vi "AlliGator Image Profile Menu Check Marks.vi"(8 "Error In":errorcluster, 11 "Menu in":refnum<k9>) -> (0 "Error Out":errorcluster)   [LabVIEW 2021, in "AlliGator Image Profile Window.lvlib"]
doc: "Handles checked items in Profile Window menu."
uses:
  AlliGator Image Profile Window.lvlib
  AlliGator Variables List.ctl
  Image/Box Profile Type.ctl
  AlliGator Image Profile Intensity Type.ctl
  AlliGator Image Profile Average Intensity Type.ctl
  Variant/Variant to Data/Variant to Boolean.vi
  AlliGator Globals, Variables & Constants.lvlib
  Variant/Variant to Data/Variant to Data.lvlib
  Image/Image.lvlib
panel:
  # "see the AlliGator License on the block diagram (Ctrl+E or Window:Show Block Diagram)"
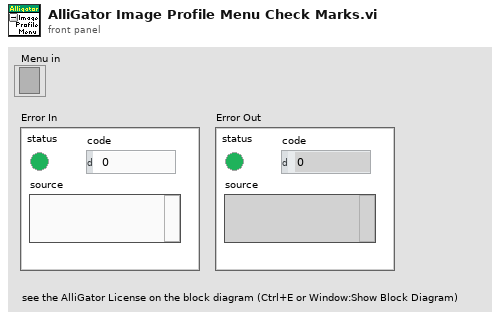
[diagram p1: front panel]
types:
  T1 = typedef "AlliGator Image Profile Window.lvlib/AlliGator Image Profile Average Intensity Type.ctl" = enum16{"Integrated Intensity", "Average Intensity", "Intensity-weighted Average Intensity"}
  T2 = typedef "AlliGator Image Profile Window.lvlib/AlliGator Image Profile Intensity Type.ctl" = enum16{"Raw Data", "Displayed Image", "Background-subtracted"}
  T3 = typedef "AlliGator Globals, Variables & Constants.lvlib/AlliGator Variables List.ctl" = enum16{"---- GUI ----", "Initialization Status", "State Indicators Refnum", "Original AlliGator Menu Items", "Current Action Loop State", "Script in progress", "Playback", "Loop Playback", "Search ROI Used", "Search ROI", "Decay Graph Max Legend Size", "Intensity Graph Max Legend Size", "Decay Statistics Graph Max Legend Size", "Phasor Graph Max Legend Size", "Phasor Ratio Graph Max Legend Size", "Lifetime Graph Max Legend Size", "---- Files ----", "Export Dataset Frames as Individual Files", "Show Batch Export Help Balloons", "Frames in Dataset", "ptu File Frame Start Indices", "Current Frame in Dataset", "Current Frame Timestamp", "------ Python Plugins ------", "Python Plugins Information", "Python Session", "Valid Python Session?", "---- Source Image ----", "Dataset Loaded", "Dataset Metadata", "Dataset Channel", "Dataset Data Description", "Background Dataset Metadata", "Background Dataset Channel", "Background Dataset Data Description", "Background File Subtraction", "Background File Path", "Background File Pile-up Correction", "Background File Pixel Well Capacity", "Background File Scaling Factor", "Source Image ROIs", "Current Source Image ROI", "Source Image ROI Event Refnum", "X_Source Image Display Range", "X_Source Image Palette Information", "Source Image Palette List", "Source Image Scale", "Current Dataset Load Settings", "Source Image:ROI Overlay Color", "---- Image Profile Window ----", "Image Profile:Overlay ROI in Source Image", "Image Profile Window Event Refnum", "Image Profile:IntensityType", "Image Profile:Intensity Average Type", "Image Profile:Intensity-weighted SDV", "Image Profile:Box Profile Type", "Image Profile Window Open", "Image Profile:Plotted Fit Parameter", "X_Type of Displayed Image", "X_Time Gate Slider", "Dataset Path", "Source Image Overlay to Erase", "Is Displayed Image Accumulated", "White Light Image Modified", "Mask Image Modified", "Macrotime Gate Separation", "------ Phasor Graph -------", "Phasor Graph:Show Line", "---- Phasor Plot ---", "Phasor Plot Parameters Changed", "FLI Dataset Modified since last Phasor Plot Calculation", "Phasor Harmonics Data", "Selected Phasor Harmonics", "Phasor Harmonic Manager Event Refnum", "Phasor Plot ROIs", "Current Phasor Plot ROI", "Phasor Plot ROI Event Refnum", "Phasor Plot Image Reference Points", "Phasor Plot Computed", "Phasor Plot Palette Information", "Phasor Plot Palette List", "Phasor Ratio Palette Information", "Phasor Ratio Palette List", "Phasor Image Scale", "Phasor Plot Image Overlay to Erase", "Phasor Plot Image Elements to Update", "Current Phasor Plot Calculation Parameters", "Current Phasor Calibration Options", "Reset Cumulated Phasor Plot", "Phasor Ratio Reference 1", "Phasor Ratio Lifetime Reference 1", "Phasor Ratio Reference 1 Frequency", "Phasor Ratio Reference 2", "Phasor Ratio Lifetime Reference 2", "Phasor Ratio Reference 2 Frequency", "---- Decay Analysis ----", "Number of Selected Decays to Fit", "LS Fit Results", "LAR Fit Results", "BS Fit Results", "Last Decay Max - Min", "Best Fit Parameters", "Best Fit Parameter Names", "Actual Size X", "Actual Size Y", "Binning X", "Binning Y", "Actual # Gates", "Dataset Number", "Gates to...", "Gates Skipped", "Gates to keep", "Gate Step", "Gate Separation", "Reversed Gates", "Pile-up Correction", "Pixel Well Capacity", "Background Subtracted", "Background Subtraction Method", "Background Definition Range", "Background File (deprecated)", "Number of Dataset Accumulated", "Array of Accumulated Dataset Paths", "Do Averaged Datasets", "Destination File Path", "Process Plot Target", "Use 1/D as Phasor Frequency", "---- Decay Fit Parameter Map -----", "Decay Fit Parameter Map Palette Information", "Decay Fit Parameter Map Palette List", "Local Decay Graph Window Event Refnum", "------- Local Decay Window ---------", "Use normalized IRF for convolution", "----- Miscellaneous ----", "Skippable Dialog Windows Status"}
  T4 = typedef "Image.lvlib/Box Profile Type.ctl" = enum16{"Full Width", "Half Width"}
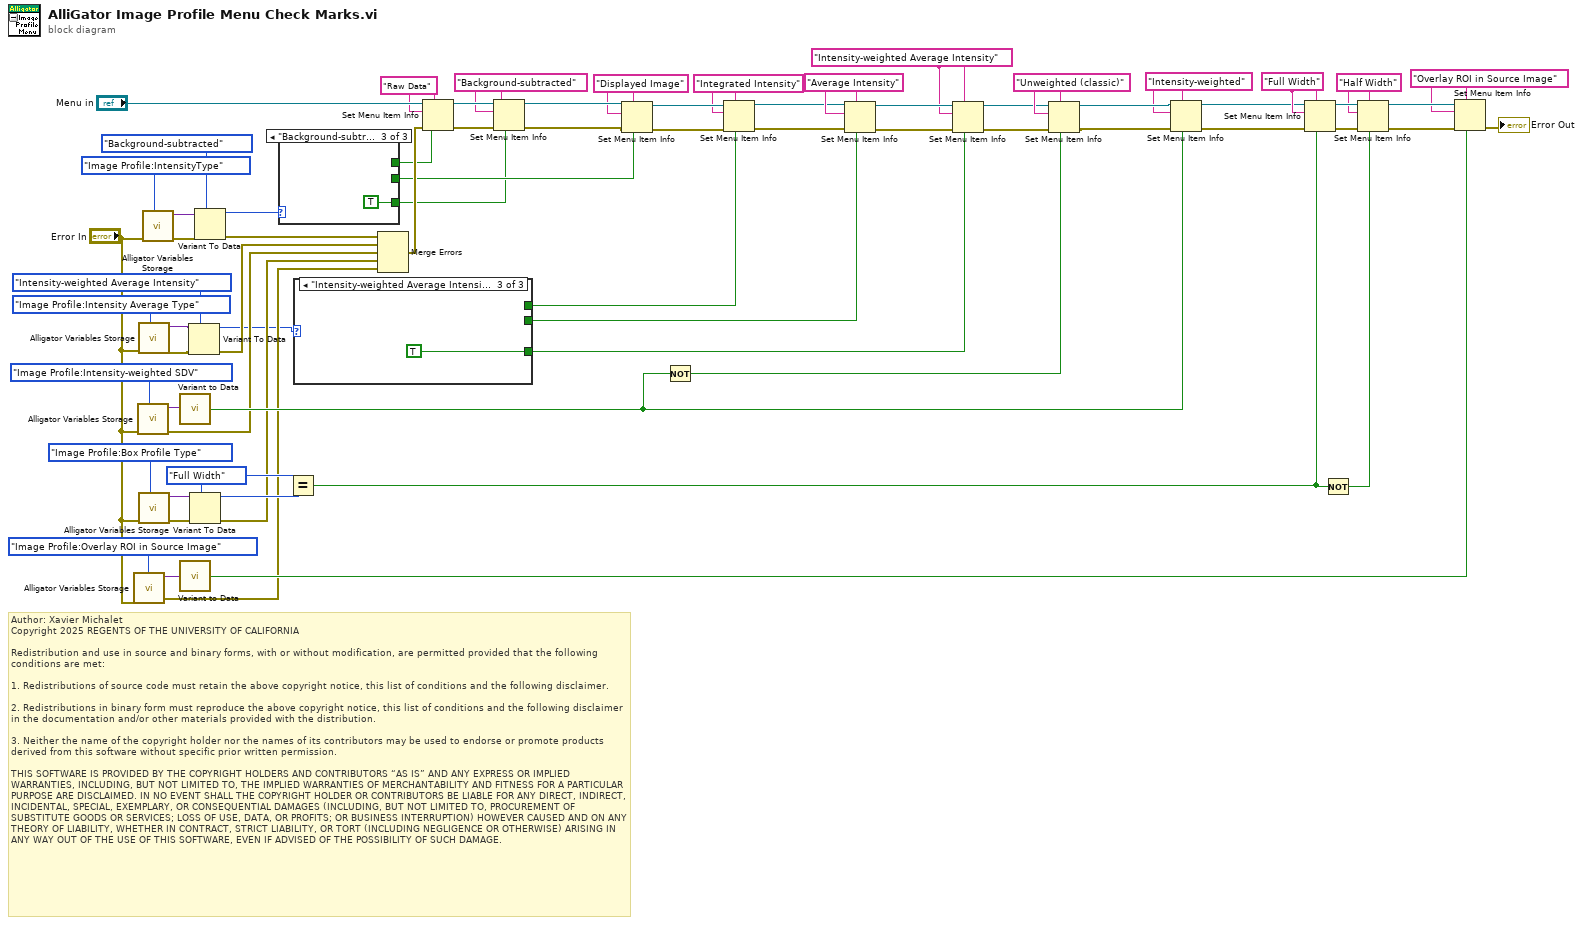
[diagram p0: block diagram]
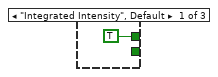
[diagram p2: hidden frame]
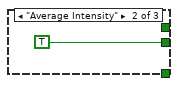
[diagram p3: hidden frame]
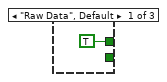
[diagram p4: hidden frame]
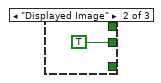
[diagram p5: hidden frame]
diagram:
  w2 = "Integrated Intensity" ("ItemTag")
  w9 = "Intensity-weighted Average Intensity" ("ItemTag")
  w10 = "Average Intensity" ("ItemTag")
  w30 = "Overlay ROI in Source Image" ("item tag")
  w46 = "Half Width" ("item tag")
  w44 = "Full Width" ("item tag")
  w48 = Box_Profile_Type."Full Width"
  w53 = "Intensity-weighted" ("ItemTag")
  w58 = "Unweighted (classic)" ("ItemTag")
  w61 = "Displayed Image" ("ItemTag")
  w65 = "Background-subtracted" ("ItemTag")
  w67 = "Raw Data" ("ItemTag")
  # "Author: Xavier Michalet\nCopyright 2025 REGENTS OF THE UNIVERSITY OF CALIFORNIA\n\nRedistribution and use in source and binary forms, with or without modification, are permitted provided that the following conditions are met:\n\n1. Redistributions of source code must retain the above copyright notice, this list of conditions and the following disclaimer.\n\n2. Redistributions in binary form must reproduce the above copyright notice, this list of conditions and the following disclaimer in the documentation and/or other materials provided with the distribution.\n\n3. Neither the name of the copyright holder nor the names of its contributors may be used to endorse or promote products derived from this software without specific prior written permission.\n\nTHIS SOFTWARE IS PROVIDED BY THE COPYRIGHT HOLDERS AND CONTRIBUTORS “AS IS” AND ANY EXPRESS OR IMPLIED WARRANTIES, INCLUDING, BUT NOT LIMITED TO, THE IMPLIED WARRANTIES OF MERCHANTABILITY AND FITNESS FOR A PARTICULAR PURPOSE ARE DISCLAIMED. IN NO EVENT SHALL THE COPYRIGHT HOLDER OR CONTRIBUTORS BE LIABLE FOR ANY DIRECT, INDIRECT, INCIDENTAL, SPECIAL, EXEMPLARY, OR CONSEQUENTIAL DAMAGES (INCLUDING, BUT NOT LIMITED TO, PROCUREMENT OF SUBSTITUTE GOODS OR SERVICES; LOSS OF USE, DATA, OR PROFITS; OR BUSINESS INTERRUPTION) HOWEVER CAUSED AND ON ANY THEORY OF LIABILITY, WHETHER IN CONTRACT, STRICT LIABILITY, OR TORT (INCLUDING NEGLIGENCE OR OTHERWISE) ARISING IN ANY WAY OUT OF THE USE OF THIS SOFTWARE, EVEN IF ADVISED OF THE POSSIBILITY OF SUCH DAMAGE."
  n1 = call "Alligator Variables Storage.vi"("AlliGator Variable"=AlliGator_Variables_List."Image Profile:Overlay ROI in Source Image" ("Alligator Variable"), "Error In"="Error In") -> ("Error Out"=w31:errorcluster, "Data out"=w36:variant)  [unwired: 7 in, 1 out]
  n2 = call "Alligator Variables Storage.vi"("AlliGator Variable"=AlliGator_Variables_List."Image Profile:Intensity-weighted SDV" ("Alligator Variable"), "Error In"="Error In") -> ("Error Out"=w38:errorcluster, "Data out"=w59:variant)  [unwired: 7 in, 1 out]
  n3 = call "Alligator Variables Storage.vi"("AlliGator Variable"=AlliGator_Variables_List."Image Profile:Intensity Average Type" ("Alligator Variable"), "Error In"="Error In") -> ("Error Out"=w19:errorcluster, "Data out"=w18:variant)  [unwired: 7 in, 1 out]
  n4 = call "Alligator Variables Storage.vi"("AlliGator Variable"=AlliGator_Variables_List."Image Profile:Box Profile Type" ("Alligator Variable"), "Error In"="Error In") -> ("Error Out"=w50:errorcluster, "Data out"=w51:variant)  [unwired: 7 in, 1 out]
  n5 = call "Alligator Variables Storage.vi"("AlliGator Variable"=AlliGator_Variables_List."Image Profile:IntensityType" ("Alligator Variable"), "Error In"="Error In") -> ("Error Out"=w26:errorcluster, "Data out"=w27:variant)  [unwired: 7 in, 1 out]
  n6 = call-poly "Variant to Data.vi"("Variant"=w59) -> ("Value"=w55:bool)  [unwired: 8 in]
  n7 = call-poly "Variant to Data.vi"("Variant"=w36) -> ("Value"=w32:bool)  [unwired: 8 in]
  n8 = Variant To Data(error in=w19, type=AlliGator_Image_Profile_Average_Intensity_Type."Intensity-weighted Average Intensity" ("Image Profile Average Intenisty Type"), Variant=w18) -> (data=w15:T1, error out=w17:errorcluster)
  n9 = Variant To Data(error in=w50, type=w48, Variant=w51) -> (data=w49:T4, error out=w37:errorcluster)
  n10 = Variant To Data(error in=w26, type=AlliGator_Image_Profile_Intensity_Type."Background-subtracted" ("Image Profile Intensity Type"), Variant=w27) -> (data=w23:T2, error out=w25:errorcluster)
  n11 = case shown="\"Background-subtracted\"" w23 {
    tunnel: [TRUE _ _] -> w22
    tunnel: [_ TRUE _] -> w21
    tunnel: [_ _ TRUE] -> w20
    frame "Raw Data", Default {
    }
    frame "Displayed Image" {
    }
    frame "Background-subtracted" {
    }
  }
  n12 = Equal?(x=w48, y=w49) -> (x = y?=w41:bool)
  n13 = case shown="\"Intensity-weighted Average Intensity\"" w15 {
    tunnel: [_ TRUE _] -> w8
    tunnel: [_ _ TRUE] -> w7
    tunnel: [TRUE _ _] -> w1
    frame "Integrated Intensity", Default {
    }
    frame "Average Intensity" {
    }
    frame "Intensity-weighted Average Intensity" {
    }
  }
  n14 = Merge Errors(w25, w17, w38, w37, w31) -> (w39:errorcluster)
  n15 = Set Menu Item Info(6:w22, 7:w67, 8:w39, 10:w67, 11:"Menu in") -> (0:w64:errorcluster, 3:w66:refnum<k9>)  [unwired: 2 in]
  n16 = Set Menu Item Info(6:w20, 7:w65, 8:w64, 10:w65, 11:w66) -> (0:w62:errorcluster, 3:w63:refnum<k9>)  [unwired: 2 in]
  n17 = Set Menu Item Info(6:w21, 7:w61, 8:w62, 10:w61, 11:w63) -> (0:w6:errorcluster, 3:w4:refnum<k9>)  [unwired: 2 in]
  n18 = Not(x=w55) -> (.not. x?=w54:bool)
  n19 = Set Menu Item Info(6:w1, 7:w2, 8:w6, 10:w2, 11:w4) -> (0:w5:errorcluster, 3:w3:refnum<k9>)  [unwired: 2 in]
  n20 = Set Menu Item Info(6:w8, 7:w10, 8:w5, 10:w10, 11:w3) -> (0:w14:errorcluster, 3:w12:refnum<k9>)  [unwired: 2 in]
  n21 = Set Menu Item Info(6:w7, 7:w9, 8:w14, 10:w9, 11:w12) -> (0:w13:errorcluster, 3:w11:refnum<k9>)  [unwired: 2 in]
  n22 = Set Menu Item Info(6:w54, 7:w58, 8:w13, 10:w58, 11:w11) -> (0:w56:errorcluster, 3:w57:refnum<k9>)  [unwired: 2 in]
  n23 = Set Menu Item Info(6:w55, 7:w53, 8:w56, 10:w53, 11:w57) -> (0:w42:errorcluster, 3:w43:refnum<k9>)  [unwired: 2 in]
  n24 = Set Menu Item Info(6:w41, 7:w44, 8:w42, 10:w44, 11:w43) -> (0:w45:errorcluster, 3:w47:refnum<k9>)  [unwired: 2 in]
  n25 = Not(x=w41) -> (.not. x?=w40:bool)
  n26 = Set Menu Item Info(6:w40, 7:w46, 8:w45, 10:w46, 11:w47) -> (0:w33:errorcluster, 3:w34:refnum<k9>)  [unwired: 2 in]
  n27 = Set Menu Item Info(6:w32, 7:w30, 8:w33, 10:w30, 11:w34) -> (0:→"Error Out":errorcluster)  [unwired: 2 in, 1 out]
